vi "ep_Read Record Info.vi"(8 "error in (no error)":errorcluster, 11 "task in":T3={"file refnums"=[], "Data Object"=refnum, "config info"={"station_name"="", "rec_dev_id"="", "rev_year"=1999.0, "TT"=0, "##A"=0, "##D"=0, "analog channel info"=[], "status channel info"=[], "lf"=50.0, "nrates"=0, "samp info"=[], "initial timestamp"=timestamp(0 s since 1904-01-01), "trigger timestamp"=timestamp(0 s since 1904-01-01), "ft"=enum."Binary", "timemult"=1.0}, "public inf content"={"Source"="", "Record Type"=enum."Unknown", "Phase ID"="", "Event Description"="", "Device ID"="", "Distance of Fault"=-1.0, "Distance Unit"=enum."Miles", "Max_Current"=inf, "Min_Current"=-inf, "Max_Voltage"=inf, "Min_Voltage"=-inf, "EventNoteCount"=0, "Event Information"=[]}, "private inf content"=[], "internal buffers"={"start index"=1, "config to public inf"=enum."disabled", "static config info"="", "static file_des record inf"="", "static file_des channel inf"="", "public inf"="", "private inf"=""}} {"public inf content"."Event Information"."min sample number" max=9999999999; "public inf content"."Event Information"."max sample number" max=9999999999; "config info"."nrates" max=999; "config info"."status channel info"."Dn" min=1 max=999999; "config info"."analog channel info"."An" min=1 max=999999; "config info"."trigger timestamp" format="%<%H:%M:%S%6u\n%d/%m/%Y>T"; "config info"."initial timestamp" format="%<%H:%M:%S%6u\n%d/%m/%Y>T"; "config info"."##D" max=999999; "config info"."##A" max=999999; "config info"."TT" min=1 max=999999; "config info"."rev_year" min=1999.0 max=1999.0}) -> (0 "error out":errorcluster, 2 "record info":T1, 3 "task out":T3={"file refnums"=[], "Data Object"=refnum, "config info"={"station_name"="", "rec_dev_id"="", "rev_year"=1999.0, "TT"=0, "##A"=0, "##D"=0, "analog channel info"=[], "status channel info"=[], "lf"=50.0, "nrates"=0, "samp info"=[], "initial timestamp"=timestamp(0 s since 1904-01-01), "trigger timestamp"=timestamp(0 s since 1904-01-01), "ft"=enum."Binary", "timemult"=1.0}, "public inf content"={"Source"="", "Record Type"=enum."Unknown", "Phase ID"="", "Event Description"="", "Device ID"="", "Distance of Fault"=-1.0, "Distance Unit"=enum."Miles", "Max_Current"=inf, "Min_Current"=-inf, "Max_Voltage"=inf, "Min_Voltage"=-inf, "EventNoteCount"=0, "Event Information"=[]}, "private inf content"=[], "internal buffers"={"start index"=1, "config to public inf"=enum."disabled", "static config info"="", "static file_des record inf"="", "static file_des channel inf"="", "public inf"="", "private inf"=""}} {"public inf content"."Event Information"."min sample number" max=9999999999; "public inf content"."Event Information"."max sample number" max=9999999999; "config info"."nrates" max=999; "config info"."status channel info"."Dn" min=1 max=999999; "config info"."analog channel info"."An" min=1 max=999999; "config info"."trigger timestamp" format="%<%H:%M:%S%6u\n%d/%m/%Y>T"; "config info"."initial timestamp" format="%<%H:%M:%S%6u\n%d/%m/%Y>T"; "config info"."##D" max=999999; "config info"."##A" max=999999; "config info"."TT" min=1 max=999999; "config info"."rev_year" min=1999.0 max=1999.0}, 4 "trigger timestamp":timestamp format="%<%H:%M:%S%6u\n%d/%m/%Y>T", 6 "file format":T2=enum."Binary")   [LabVIEW 2014, in "NI_EP_COMTRADE.lvlib"]
uses:
  <vilib>/addons/Electrical Power/File IO/NI_EP_COMTRADE.lvlib
  <vilib>/addons/Electrical Power/File IO/COMTRADE/typedefs/ep_Task.ctl
  <vilib>/addons/Electrical Power/File IO/COMTRADE/typedefs/ep_Config Info.ctl
  <vilib>/addons/Electrical Power/File IO/COMTRADE/typedefs/ep_Analog Channel Info.ctl
  <vilib>/addons/Electrical Power/File IO/COMTRADE/typedefs/ep_Status Channel Info.ctl
  <vilib>/addons/Electrical Power/File IO/COMTRADE/typedefs/ep_File Format.ctl
  <vilib>/addons/Electrical Power/File IO/COMTRADE/typedefs/ep_Public Inf Content.ctl
  <vilib>/addons/Electrical Power/File IO/COMTRADE/typedefs/ep_Public Event Inf.ctl
  <vilib>/addons/Electrical Power/File IO/COMTRADE/typedefs/ep_Private Inf Content.ctl
  <vilib>/addons/Electrical Power/File IO/COMTRADE/typedefs/ep_System Record Inf.ctl
  <vilib>/Platform/storage/Storage.llb/Get Property (Storage Refnums).vi
  <vilib>/Platform/storage/Storage.llb/Get Property (String).vi
  <vilib>/Platform/storage/Storage.llb/Get Property (SGL).vi
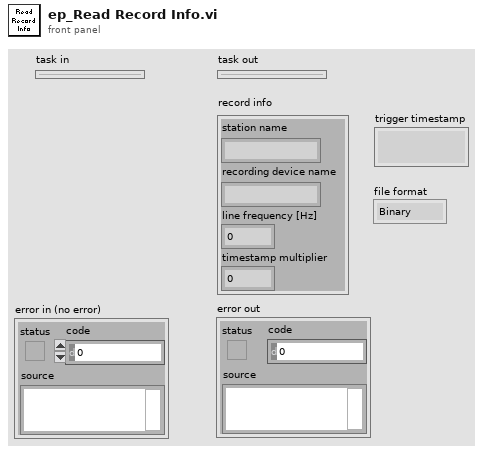
[diagram p1: front panel]
types:
  T1 = typedef "NI_EP_COMTRADE.lvlib/ep_System Record Inf.ctl" = cluster{"station name":string, "recording device name":string, "line frequency [Hz]":sgl, "timestamp multiplier":sgl}
  T2 = typedef "NI_EP_COMTRADE.lvlib/ep_File Format.ctl" = enum16{"ASCII", "Binary"}
  T3 = typedef "NI_EP_COMTRADE.lvlib/ep_Task.ctl" = cluster{"file refnums":refnum<file>[], "Data Object":refnum<k20>, "config info":T4, "public inf content":T7, "private inf content":T9, "internal buffers":cluster{"start index":u32, "config to public inf":enum16{"disabled", "enabled", "buffered"}, "static config info":string, "static file_des record inf":string, "static file_des channel inf":string, "public inf":string, "private inf":string}}
  T4 = typedef "NI_EP_COMTRADE.lvlib/ep_Config Info.ctl" = cluster{"station_name":string, "rec_dev_id":string, "rev_year":dbl, "TT":u32, "##A":u32, "##D":u32, "analog channel info":T5[], "status channel info":T6[], "lf":sgl, "nrates":u16, "samp info":cluster{"samp":sgl, "endsamp":u32}[], "initial timestamp":timestamp, "trigger timestamp":timestamp, "ft":T2, "timemult":sgl}
  T5 = typedef "NI_EP_COMTRADE.lvlib/ep_Analog Channel Info.ctl" = cluster{"An":u32, "ch_id":string, "ph":string, "ccbm":string, "uu":string, "a":sgl, "b":sgl, "skew":sgl, "min":i32, "max":i32, "primary":sgl, "secondary":sgl, "PS":enum16{"P", "S"}}
  T6 = typedef "NI_EP_COMTRADE.lvlib/ep_Status Channel Info.ctl" = cluster{"Dn":u32, "ch_id":string, "ph":string, "ccbm":string, "Y":bool}
  T7 = typedef "NI_EP_COMTRADE.lvlib/ep_Public Inf Content.ctl" = cluster{"Source":string, "Record Type":enum16{"Fault", "Unknown", "Misoperation", "Close", "Trip", "Reclose", "Power swing", "Simulation"}, "Phase ID":string, "Event Description":string, "Device ID":string, "Distance of Fault":dbl, "Distance Unit":enum16{"Miles", "Kilometers", "Percent of line", "Percent of setting", "Ohms"}, "Max_Current":dbl, "Min_Current":dbl, "Max_Voltage":dbl, "Min_Voltage":dbl, "EventNoteCount":u32, "Event Information":T8[]}
  T8 = typedef "NI_EP_COMTRADE.lvlib/ep_Public Event Inf.ctl" = cluster{"channel number":u32, "max value":dbl, "min value":dbl, "max sample number":u64, "min sample number":u64, "max sample text":string[], "min sample text":string[]}
  T9 = typedef "NI_EP_COMTRADE.lvlib/ep_Private Inf Content.ctl" = cluster{"Section Header":string, "Entry Names":string[], "Entry Values":string[]}[]
  T10 = cluster{"Value":string, "Value":string, "Value":sgl, "Value":sgl}
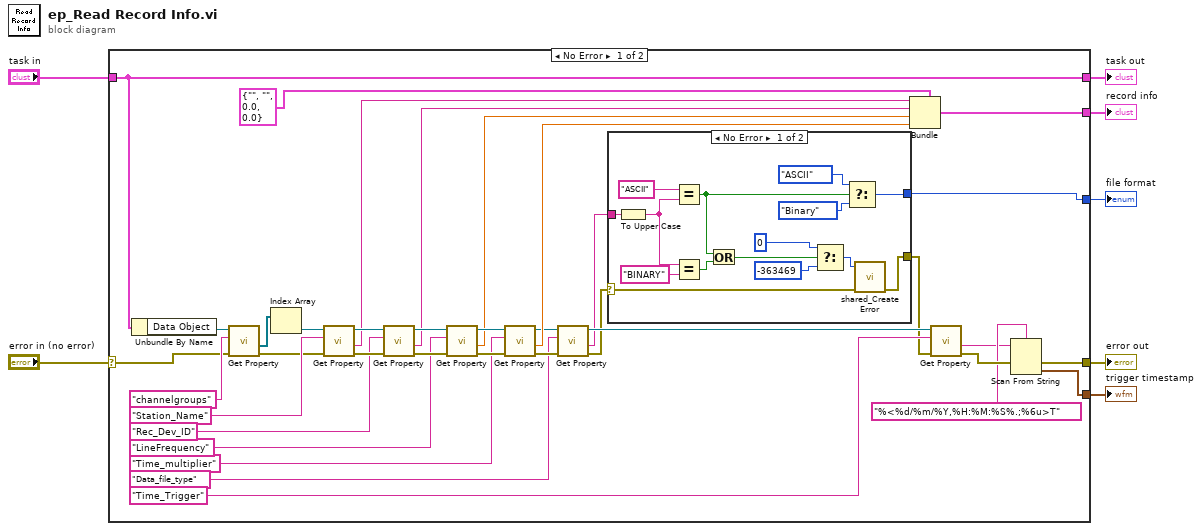
[diagram p0: block diagram]
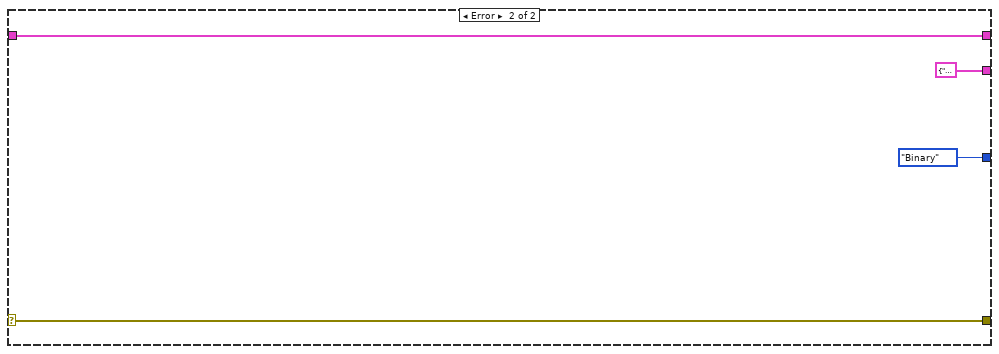
[diagram p3: hidden frame]
diagram:
  n1 = case shown="No Error" "error in (no error)" {
    selector: "error in (no error)" -> [w20 w63]
    tunnel: "task in" -> [w19 w64]
    tunnel: [w19 w64] -> w5
    tunnel: [w8 enum16{"ASCII", "Binary"}."Binary" ("file format")] -> w4
    tunnel: [w18 T10 {"Value"="", "Value"="", "Value"=0.0, "Value"=0.0}] -> w3
    tunnel: [w15 _] -> w2
    tunnel: [w14 w63] -> w1
    frame No Error {
      n2 = Unbundle By Name(w19) -> ("Data Object"=w44:refnum<k20>)
      n3 = call-poly <vilib>:"Get Property.vi"("error in (no error)"=w20, "Property name"="channelgroups", "storage refnum"=w44) -> ("error out"=w40:errorcluster, "Value"=w42:refnum<k20>[])  [unwired: 6 in, 1 out]
      n4 = Index Array(array=w42) -> (element=w22:refnum<k20>)  [unwired: 1 in]
      n5 = call-poly <vilib>:"Get Property.vi"("error in (no error)"=w40, "Property name"="Station_Name", "storage refnum"=w22) -> ("error out"=w39:errorcluster, "Value"=w30:string, "storage refnum out"=w38:refnum<k20>)  [unwired: 6 in]
      n6 = call-poly <vilib>:"Get Property.vi"("error in (no error)"=w39, "Property name"="Rec_Dev_ID", "storage refnum"=w38) -> ("error out"=w36:errorcluster, "Value"=w29:string, "storage refnum out"=w35:refnum<k20>)  [unwired: 6 in]
      n7 = call-poly <vilib>:"Get Property.vi"("error in (no error)"=w36, "Property name"="LineFrequency", "storage refnum"=w35) -> ("error out"=w33:errorcluster, "Value"=w28:sgl, "storage refnum out"=w32:refnum<k20>)  [unwired: 6 in]
      n8 = call-poly <vilib>:"Get Property.vi"("error in (no error)"=w33, "Property name"="Time_multiplier", "storage refnum"=w32) -> ("error out"=w25:errorcluster, "Value"=w27:sgl, "storage refnum out"=w26:refnum<k20>)  [unwired: 6 in]
      n9 = call-poly <vilib>:"Get Property.vi"("error in (no error)"=w25, "Property name"="Data_file_type", "storage refnum"=w26) -> ("error out"=w11:errorcluster, "Value"=w9:string, "storage refnum out"=w24:refnum<k20>)  [unwired: 6 in]
      n10 = case shown="No Error" w11 {
        selector: w11 -> [w49 w60]
        tunnel: [w45 w60] -> w10
        tunnel: w9 -> [w59 _]
        tunnel: [w51 _] -> w8
        frame No Error {
          n11 = To Upper Case(1:w59) -> (0:w56:string)
          n12 = Equal?(x="ASCII" ("y"), y=w56) -> (x = y?=w53:bool)
          n13 = Equal?(x=w56, y="BINARY") -> (x = y?=w52:bool)
          n14 = Or(x=w53, y=w52) -> (x .or. y?=w50:bool)
          n15 = Select(t=0 ("error code (0)"), s=w50, f=-363469 ("error code (0)")) -> (s? t:f=w46:i32)
          n16 = Select(t=ep_File_Format."ASCII" ("file format"), s=w53, f=ep_File_Format."Binary") -> (s? t:f=w51:T2)
          n17 = call <vilib>:"shared_Create Error.vi"("error in (no error)"=w49, "error code (0)"=w46) -> ("error out"=w45:errorcluster)  [unwired: 9 in]
        }
        frame Error {
        }
      }
      n18 = Bundle(cluster=T1 {"station name"="", "recording device name"="", "line frequency [Hz]"=0.0, "timestamp multiplier"=0.0}, "station name"=w30, "recording device name"=w29, "line frequency [Hz]"=w28, "timestamp multiplier"=w27) -> (w18:T1)
      n19 = call-poly <vilib>:"Get Property.vi"("error in (no error)"=w10, "Property name"="Time_Trigger", "storage refnum"=w24) -> ("error out"=w17:errorcluster, "Value"=w13:string)  [unwired: 6 in, 1 out]
      n20 = Scan From String(format string="%<%d/%m/%Y,%H:%M:%S%.;%6u>T", input string=w13, error in=w17) -> (error out=w14:errorcluster, output 1=w15:timestamp)  [unwired: 2 in, 2 out]
    }
    frame Error {
    }
  }
  "task out" <- w5
  "trigger timestamp" <- w2
  "file format" <- w4
  "record info" <- w3
  "error out" <- w1
